vi "supercontinuumControl.vi"() -> ()   [LabVIEW 2011]
uses:
  monochromatorcontrol/perHandlemonochromator.vi
  users/nicolas/PHySpec-SDK-1.0.0/Labview-example/libPhyspec/libPhyspec.lvlib
panel:
  in  "readout rate (ms)":i32=2000 max=0
  in  "pm100usb":bool
  out "Laser power (µW)":dbl
  in  "RFonoff":bool
  in  "PortParameters":T1={"OpenPort"=TRUE, "ClosePort"=FALSE, "Baudrate"=115200, "Wait"=50, "ReadWrite"=FALSE}
  in  "InParameters":T2={"Destination"=18, "Source"=162, "Register"=144, "Array"=[], "WriteNotRead"=FALSE, "ReadWithPreample"=FALSE, "Ring"=3, "String"="", "Long"=0} {"Ring" items=["ByteArray", "IntegerArray", "String", "Long", "Direct string sent"]; "Register" format="%x"}
  out "peHandle":u32
  out "final error":errorcluster
  in  "Amplitude\nCH3 (%)":dbl=800.0 min=800.0 max=1400.0 step=1.0 format="%#.3g"
  in  "CH3 (nm)":dbl=800.0 min=800.0 max=1400.0 step=1.0 format="%#.3g"
  in  "Amplitude\nCH2 (%)":dbl=800.0 min=0.0 max=1400.0 step=0.1 format="%#.3g"
  in  "CH2 (nm)":dbl=800.0 min=800.0 max=1400.0 step=1.0 format="%#.3g"
  in  "Amplitude\nCH1 (%)":dbl=100.0 min=0.0 max=100.0 step=0.1 format="%#.3g"
  in  "CH1 (nm)":dbl=800.0 min=800.0 max=1400.0 step=1.0 format="%#.3g"
  in  "Amplitude\nCH0 (%)":dbl=100.0 min=0.0 max=100.0 step=0.1 format="%#.1f"
  in  "EXIT":bool
  in  "stop NKT  select":bool
  in  "CH0 (nm)":dbl=800.0 min=800.0 max=1400.0 step=1.0 format="%#.3g"
  in  "stop lttf":bool
  out "Current wavelength (nm)":dbl
  in  "SET wavelength (nm)":dbl max=0.0
  in  "NKT COM port":refnum<visa-resource-name>="COM21"
  out "NKT select":bool
  in  "NKT select start":bool
  out "LTTF contrast":bool
  in  "start LTTF filter":bool
  out "Fianium connected":bool
  in  "start fianium":bool
  out "Alarm":i32
  out "Output":string
  in  "Custom command":string
  out "Back Reflection Monitor":i32
  out "appended array":bool[](array[boolean])
  in  "100percent":bool
  in  "75percent":bool
  in  "50percent":bool
  in  "25percent":bool
  in  "power 0":bool
  in  "Set Power":i32 max=2100
  out "Power":i32
  out "Current Power":u8(slide) scale=0.0..100.0
  out "max Q":i32
  out "error out":errorcluster
  in  "Fianium COM port":refnum<visa-resource-name>="COM19"
  out "MachineState":string="init"
  in  "KEY":bool
  in  "stop fianium":bool
  # "Fianium WL-SC400 control"
  # "SET POWER"
  # "PM100"
  # "NKT Select"
  # "LTTF contrast"
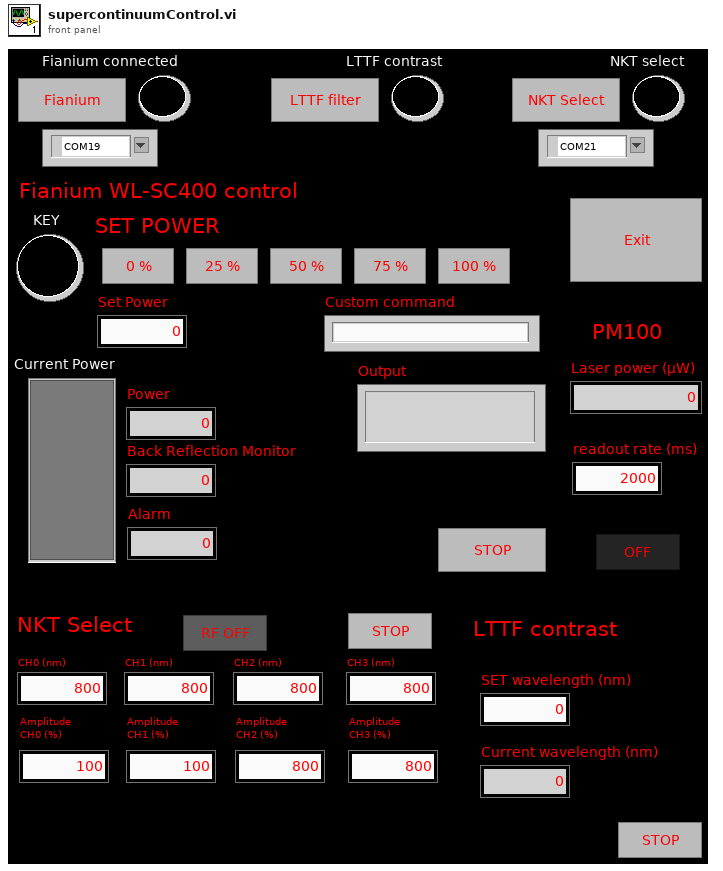
[diagram p1: front panel]
types:
  T1 = cluster{"OpenPort":bool, "ClosePort":bool, "Baudrate":i32, "Wait":u16, "ReadWrite":bool}
  T2 = cluster{"Destination":u8, "Source":u8, "Register":u8, "Array":i16[], "WriteNotRead":bool, "ReadWithPreample":bool, "Ring":u16, "String":string, "Long":i32}
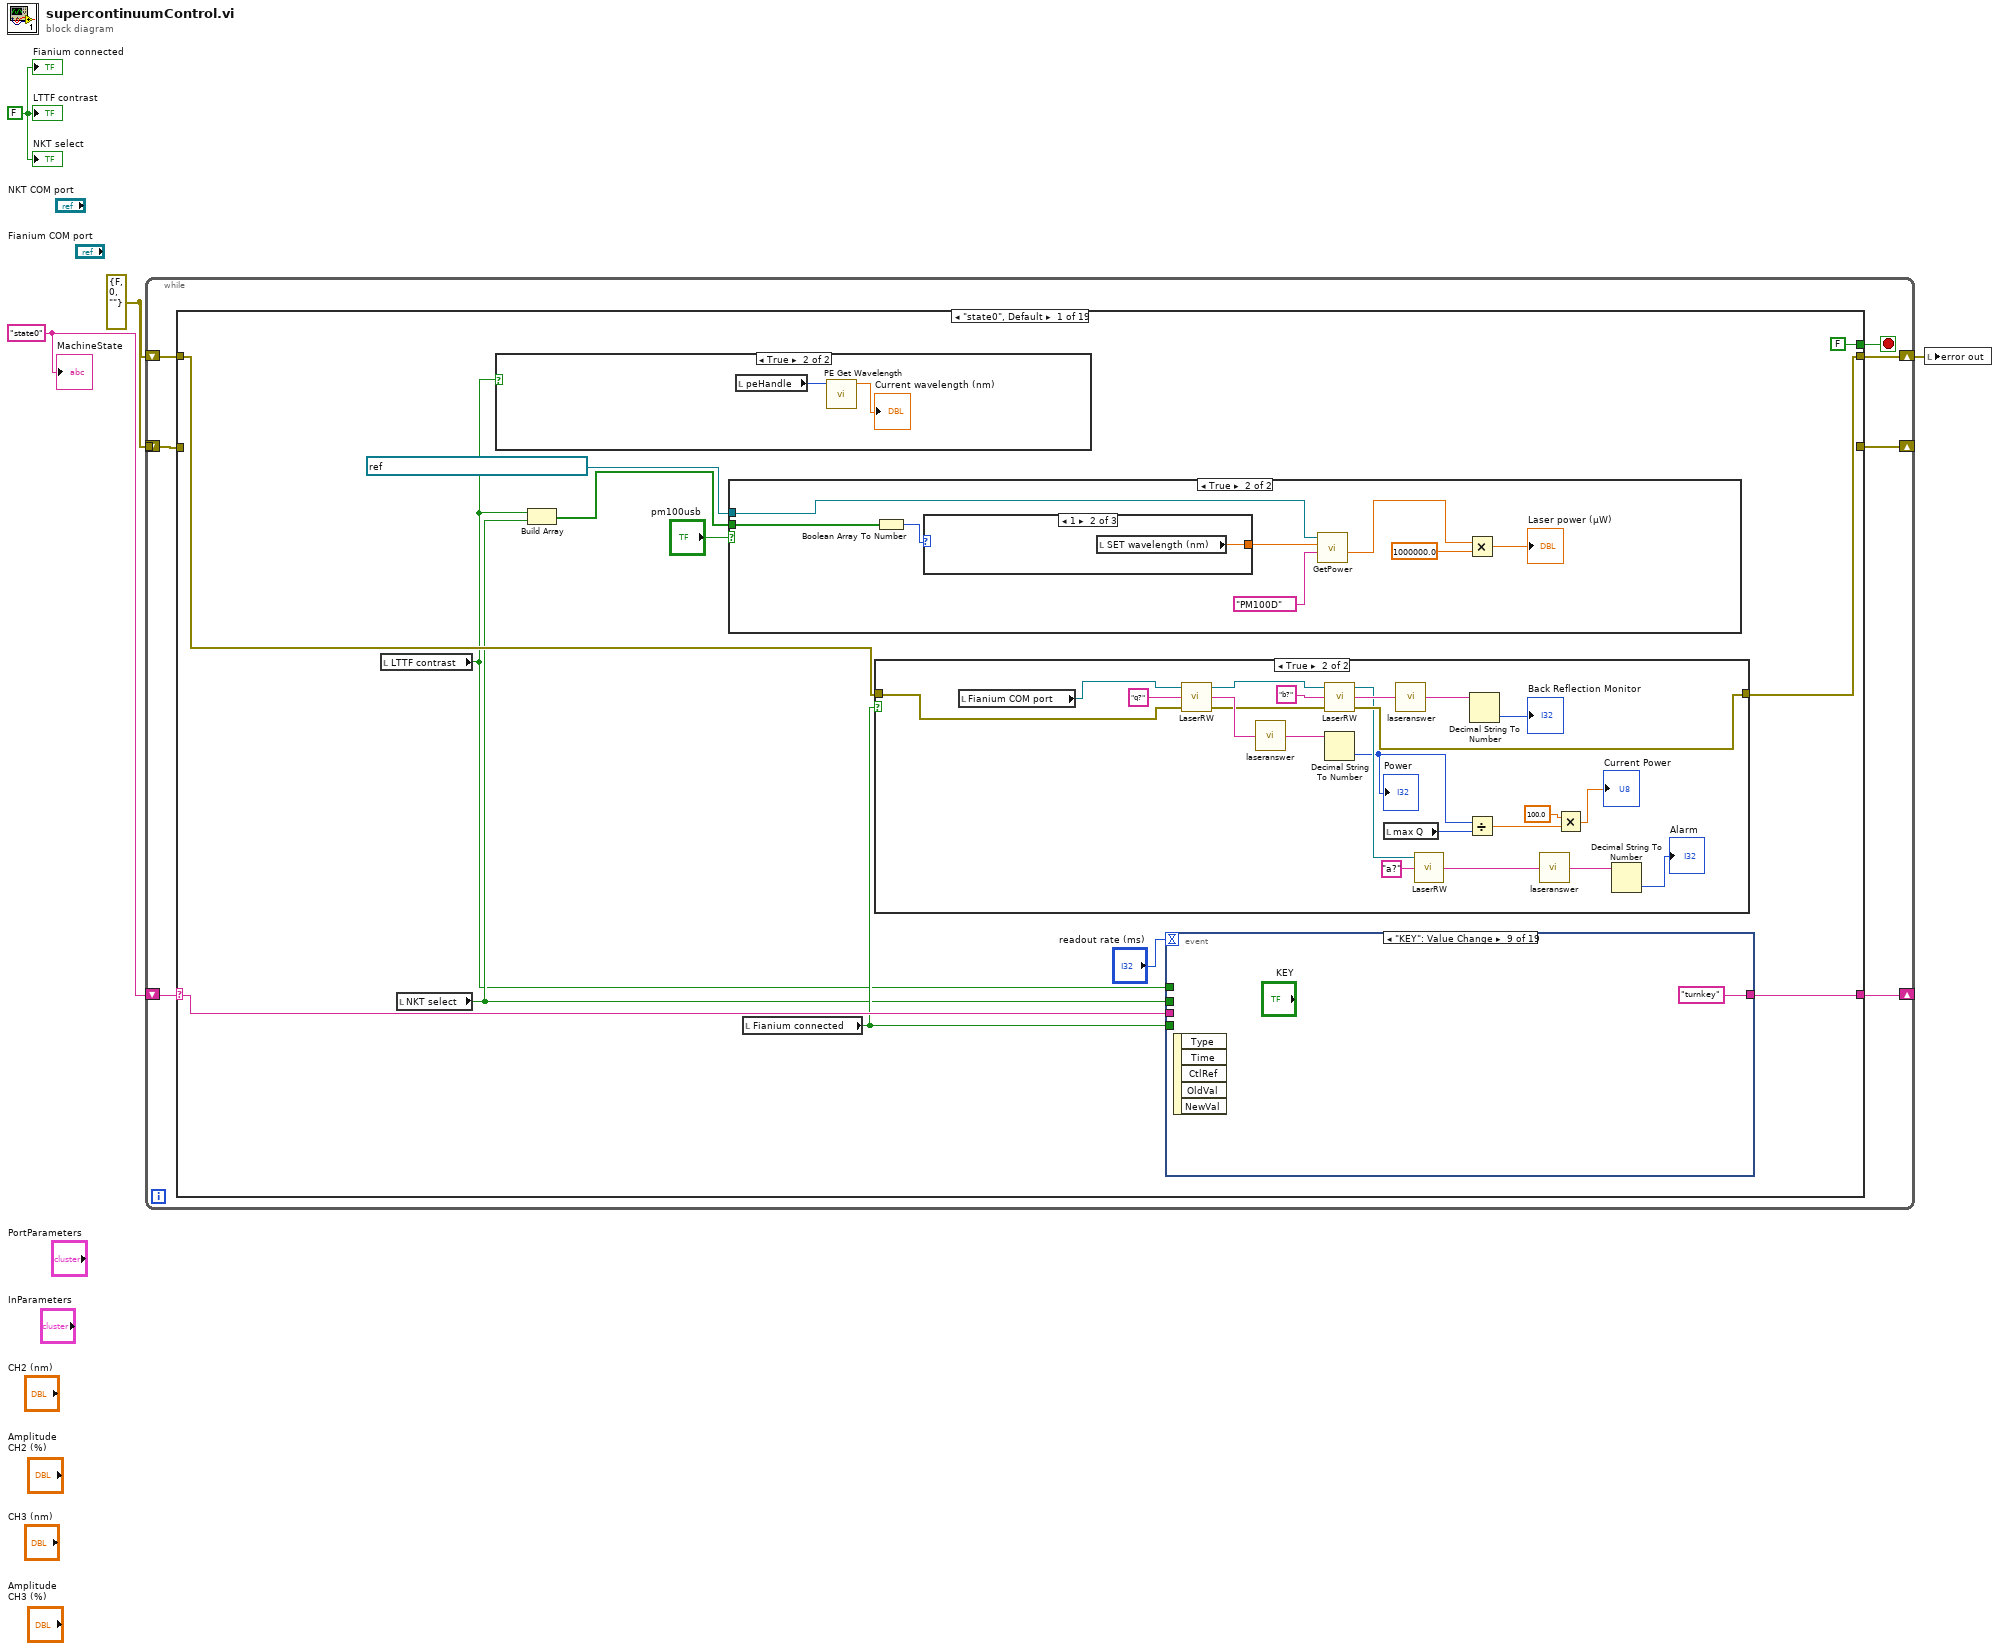
[diagram p0: block diagram]
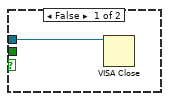
[diagram p2: hidden frame]
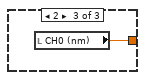
[diagram p4: hidden frame]
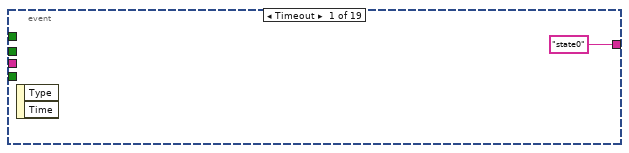
[diagram p7: hidden frame]
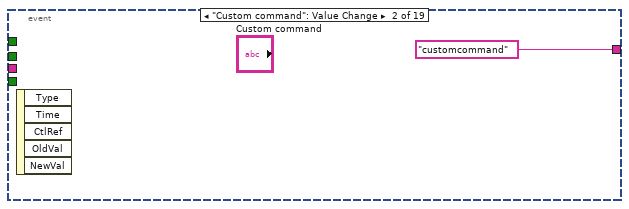
[diagram p8: hidden frame]
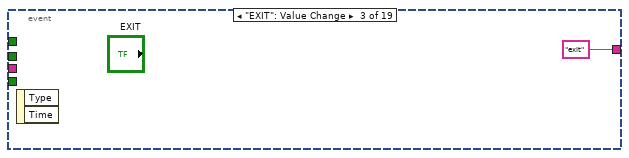
[diagram p9: hidden frame]
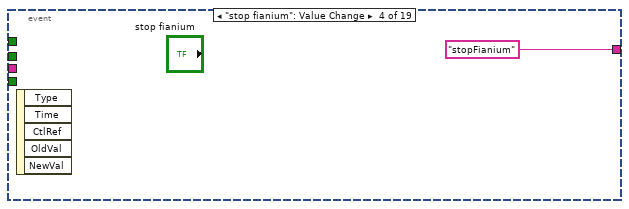
[diagram p10: hidden frame]
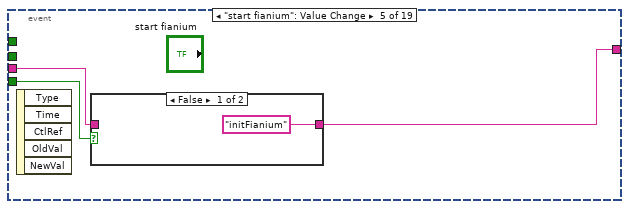
[diagram p11: hidden frame]
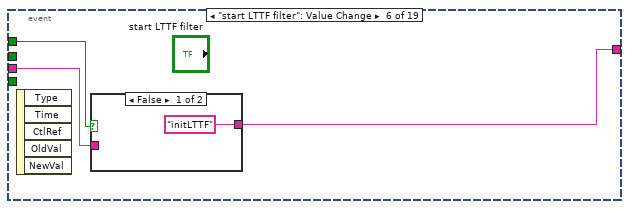
[diagram p13: hidden frame]
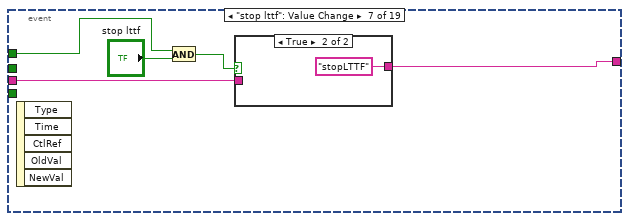
[diagram p15: hidden frame]
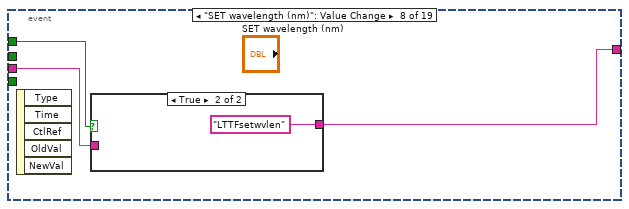
[diagram p17: hidden frame]
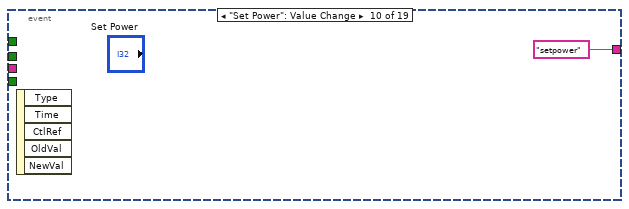
[diagram p19: hidden frame]
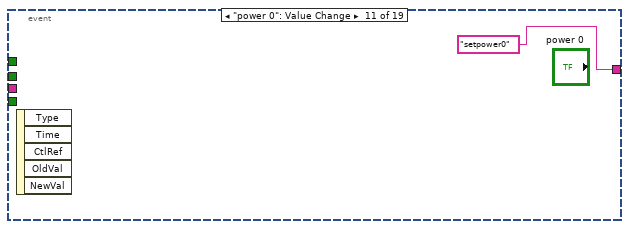
[diagram p20: hidden frame]
diagram:
  w2 = FALSE
  w1 = errorcluster {"status"=FALSE, "code"=0, "source"=""} ("error out")
  w4 = "state0"
  n1 = while {
    shift-right: [w10] -> _
    shift-left: w4 -> [w11]
    shift-right: [w8] -> w3
    shift-left: w1 -> [w7]
    shift-right: [w5] -> _
    shift-left: w1 -> [w6]
    tunnel: [w6] -> _
    stop <- w9 stop-if-true
    n2 = case shown="\"state0\", Default" w11 {
      selector: w11 -> [w19 _ _ _ _ _ _ _ _ _ _ _ _ _ _ _ _ _ _]
      tunnel: [w23 "state0" "state0" "state0" "" "state0" "state0" "state0" "state0" "state0" "state0" "state0" "state0" "state0" "state0" "state0" "state0" "state0" "state0"] -> w10
      tunnel: [FALSE _ _ _ TRUE FALSE FALSE FALSE FALSE FALSE _ FALSE _ _ _ _ _ _ _] -> w9
      tunnel: [w21 _ _ _ w167 w172 w180 w211 w216 w225 w244 w265 w282 w293 w302 w318 w335 w352 w378] -> w8
      tunnel: w7 -> [w22 _ _ _ w167 w173 w179 w212 w223 w227 w248 w267 w282 w293 w302 w318 w335 w352 w378]
      tunnel: w6 -> [_ w130 w149 w157 _ _ _ _ _ _ _ _ _ _ _ _ _ _ _]
      tunnel: [_ w131 w148 w156 _ _ _ _ _ _ _ _ _ _ _ _ _ _ _] -> w5
      frame "state0", Default {
        n3 = local read "LTTF contrast"() -> (w15:bool)
        n4 = local read "NKT select"() -> (w16:bool)
        n5 = case shown="True" w15 {
          frame False {
          }
          frame True {
            n6 = local read "peHandle"() -> (w35:u32)
            n7 = call "PE Get Wavelength.vi"("peHandle"=w35) -> ("wavelength"=→"Current wavelength (nm)":dbl)  [unwired: 8 in, 2 out]
          }
        }
        n8 = Build Array(w15, w16) -> (w13:bool[])
        n9 = case shown="True" "pm100usb" {
          tunnel: refnum<visa-resource-name> "USB0::0x1313::0x8072::P2007928::INSTR" ("Input Device") -> [w24 w31]
          tunnel: w13 -> [_ w28]
          frame False {
            n10 = VISA Close(VISA resource name=w24) -> ()  [unwired: 1 in, 1 out]
          }
          frame True {
            n11 = Boolean Array To Number(Boolean array=w28) -> (number=w27:u32)
            n12 = case shown="1" w27 {
              tunnel: [_ w33 w34] -> w26
              frame 0, Default {
              }
              frame 1 {
                n13 = local read "SET wavelength (nm)"() -> (w33:dbl)
              }
              frame 2 {
                n14 = local read "CH0 (nm)"() -> (w34:dbl)
              }
            }
            n15 = call "GetPower.vi"("Measeaurement mode"="PM100D", "Wavelength (nm)"=w26, "Input Device"=w31) -> ("Power (W)"=w30:dbl)  [unwired: 1 in, 3 out]
            n16 = Multiply(x=w30, y=1000000.0) -> (x*y=→"Laser power (µW)":dbl)
          }
        }
        n17 = local read "Fianium connected"() -> (w18:bool)
        n18 = case shown="True" w18 {
          tunnel: w22 -> [w37 w58]
          tunnel: [w37 w46] -> w21
          frame False {
          }
          frame True {
            n19 = local read "Fianium COM port"() -> (w59:refnum<visa-resource-name>)
            n20 = call "LaserRW.vi"("error in (no error)"=w58, "buffer à écrire"="q?", "Nom de ressource VISA"=w59) -> ("error out"=w49:errorcluster, "buffer lu"=w56:string, "Nom de ressource VISA en sortie"=w50:refnum<visa-resource-name>)
            n21 = call "laseranswer.vi"("IN"=w56) -> ("Answer"=w55:string)
            n22 = call "LaserRW.vi"("error in (no error)"=w49, "buffer à écrire"="b?", "Nom de ressource VISA"=w50) -> ("error out"=w46:errorcluster, "buffer lu"=w47:string, "Nom de ressource VISA en sortie"=w44:refnum<visa-resource-name>)
            n23 = Decimal String To Number(string=w55) -> (number=w39:i32)  [unwired: 2 in, 1 out]
            "Power" <- w39
            n24 = local read "max Q"() -> (w54:i32)
            n25 = call "laseranswer.vi"("IN"=w47) -> ("Answer"=w45:string)
            n26 = call "LaserRW.vi"("buffer à écrire"="a?", "Nom de ressource VISA"=w44) -> ("buffer lu"=w38:string)  [unwired: 1 in, 2 out]
            n27 = Divide(x=w39, y=w54) -> (x/y=w53:dbl)
            n28 = Decimal String To Number(string=w45) -> (number=→"Back Reflection Monitor":i32)  [unwired: 2 in, 1 out]
            n29 = call "laseranswer.vi"("IN"=w38) -> ("Answer"=w43:string)
            n30 = Multiply(x=100.0, y=w53) -> (x*y=→"Current Power":dbl)
            n31 = Decimal String To Number(string=w43) -> (number=→"Alarm":i32)  [unwired: 2 in, 1 out]
          }
        }
        n32 = event shown="[8] \"KEY\": Value Change" {
          selector: _ -> [_ _ _ _ _ _ _ _ _ _ _ _ _ _ _ _ _ _ _]
          dyn-events: _ -> [_ _ _ _ _ _ _ _ _ _ _ _ _ _ _ _ _ _ _]
          timeout: "readout rate (ms)" -> [_ _ _ _ _ _ _ _ _ _ _ _ _ _ _ _ _ _ _]
          tunnel: ["state0" "customcommand" "exit" "stopFianium" w66 w71 w78 w82 "turnkey" "setpower" "setpower0" "percentchange" w96 w102 w106 w112 w116 w121 w126] -> w23
          tunnel: w19 -> [_ _ _ _ w65 w70 w77 w81 _ _ _ _ w95 w101 w105 w110 w115 w120 w125]
          tunnel: w18 -> [_ _ _ _ w64 _ _ _ _ _ _ _ _ _ _ _ _ _ _]
          tunnel: w15 -> [_ _ _ _ _ w69 w75 w83 _ _ _ _ _ _ _ _ _ _ _]
          tunnel: w16 -> [_ _ _ _ _ _ _ _ _ _ _ _ w97 w100 w107 w111 w117 w122 w127]
          event Timeout {
            n33 = event-data() -> ()  [unwired: 1 in, 2 out]
          }
          event "Custom command": Value Change {
            n34 = event-data() -> ()  [unwired: 1 in, 5 out]
          }
          event "EXIT": Value Change {
            n35 = event-data() -> ()  [unwired: 1 in, 2 out]
          }
          event "stop fianium": Value Change {
            n36 = event-data() -> ()  [unwired: 1 in, 5 out]
          }
          event "start fianium": Value Change {
            n37 = event-data() -> ()  [unwired: 1 in, 5 out]
            n38 = case shown="False" w64 {
              tunnel: ["initFianium" w68] -> w66
              tunnel: w65 -> [_ w68]
              frame False {
              }
              frame True {
              }
            }
          }
          event "start LTTF filter": Value Change {
            n39 = event-data() -> ()  [unwired: 1 in, 5 out]
            n40 = case shown="False" w69 {
              tunnel: ["initLTTF" w73] -> w71
              tunnel: w70 -> [_ w73]
              frame False {
              }
              frame True {
              }
            }
          }
          event "stop lttf": Value Change {
            n41 = event-data() -> ()  [unwired: 1 in, 5 out]
            n42 = And(x=w75, y="stop lttf") -> (x .and. y?=w74:bool)
            n43 = case shown="True" w74 {
              tunnel: [w79 "stopLTTF"] -> w78
              tunnel: w77 -> [w79 _]
              frame False {
              }
              frame True {
              }
            }
          }
          event "SET wavelength (nm)": Value Change {
            n44 = event-data() -> ()  [unwired: 1 in, 5 out]
            n45 = case shown="True" w83 {
              tunnel: [w84 "LTTFsetwvlen"] -> w82
              tunnel: w81 -> [w84 _]
              frame False {
              }
              frame True {
              }
            }
          }
          event "KEY": Value Change {
            n46 = event-data() -> ()  [unwired: 1 in, 5 out]
          }
          event "Set Power": Value Change {
            n47 = event-data() -> ()  [unwired: 1 in, 5 out]
          }
          event "power 0": Value Change {
            n48 = event-data() -> ()  [unwired: 1 in, 5 out]
          }
          event "25percent", "50percent", "75percent", "100percent": Value Change {
            n49 = event-data() -> ()  [unwired: 1 in, 5 out]
            n50 = Build Array("25percent", "50percent", "75percent", "100percent") -> (→"appended array":bool[])
          }
          event "NKT select start": Value Change {
            n51 = event-data() -> ()  [unwired: 1 in, 5 out]
            n52 = case shown="False" w97 {
              tunnel: ["NKTSELECTstart" w99] -> w96
              tunnel: w95 -> [_ w99]
              frame False {
              }
              frame True {
              }
            }
          }
          event "stop NKT  select": Value Change {
            n53 = event-data() -> ()  [unwired: 1 in, 5 out]
            n54 = case shown="True" w100 {
              tunnel: w101 -> [w103 _]
              tunnel: [w103 "NKTSELECTstop"] -> w102
              frame False {
              }
              frame True {
              }
            }
          }
          event "CH0 (nm)": Value Change {
            n55 = event-data() -> ()  [unwired: 1 in, 7 out]
            n56 = case shown="True" w107 {
              tunnel: [w108 "NKTSELECTch0wv"] -> w106
              tunnel: w105 -> [w108 _]
              frame False {
              }
              frame True {
              }
            }
          }
          event "Amplitude\nCH0 (%)": Value Change {
            n57 = event-data() -> ()  [unwired: 1 in, 5 out]
            n58 = case shown="True" w111 {
              tunnel: [w113 "NKTSELECTampch0"] -> w112
              tunnel: w110 -> [w113 _]
              frame False {
              }
              frame True {
              }
            }
          }
          event "RFonoff": Value Change {
            n59 = event-data() -> ()  [unwired: 1 in, 5 out]
            n60 = case shown="False" w117 {
              tunnel: [w118 "NKTselectrfonoff"] -> w116
              tunnel: w115 -> [w118 _]
              frame False {
              }
              frame True {
              }
            }
          }
          event "CH1 (nm)": Value Change {
            n61 = event-data() -> ()  [unwired: 1 in, 5 out]
            n62 = case shown="True" w122 {
              tunnel: [w123 "NKTSELECTch1wv"] -> w121
              tunnel: w120 -> [w123 _]
              frame False {
              }
              frame True {
              }
            }
          }
          event "Amplitude\nCH1 (%)": Value Change {
            n63 = event-data() -> ()  [unwired: 1 in, 5 out]
            n64 = case shown="True" w127 {
              tunnel: [w128 "NKTSELECTampch1"] -> w126
              tunnel: w125 -> [w128 _]
              frame False {
              }
              frame True {
              }
            }
          }
        }
      }
      frame "initLTTF" {
        n65 = Path To String(path=path "C:/Program Files (x86)/Photon etc/PHySpecV2/system.xml" ("Configuration File")) -> (string=w136:string)
        n66 = call "PE Create.vi"("error in (no error)"=w130, "conffile"=w136) -> ("error out"=w138:errorcluster, "peHandle"=w137:u32)  [unwired: 7 in, 1 out]
        n67 = case shown="No Error" w138 {
          selector: w138 -> [w144 w147]
          tunnel: w137 -> [w141 _]
          tunnel: [w141 _] -> w134
          tunnel: [w140 w147] -> w131
          frame No Error {
            n68 = call "PE Get System Name.vi"("error in (no error)"=w144, "size"=4095, "index"=0, "peHandle"=w141) -> ("error out"=w143:errorcluster, "name"=w142:string)  [unwired: 5 in, 1 out]
            n69 = call "PE Open.vi"("error in (no error)"=w143, "name"=w142, "peHandle"=w141) -> ("error out"=w140:errorcluster)  [unwired: 7 in, 1 out]
          }
          frame Error {
          }
        }
        "peHandle" <- w134
        n70 = global write "perHandlemonochromator.vi" "peHandle"(w134) -> ()
        n71 = Unbundle By Name(w131) -> ("status"=w133:bool)
        n72 = Not(x=w133) -> (.not. x?=w132:bool)
        n73 = local write "LTTF contrast"(w132) -> ()
      }
      frame "LTTFsetwvlen" {
        n74 = local read "SET wavelength (nm)"() -> (w152:dbl)
        n75 = In Range and Coerce(upper limit=400.0, x=w152, lower limit=1100.0) -> (coerced(x)=w151:dbl)  [unwired: 1 out]
        n76 = local read "peHandle"() -> (w150:u32)
        n77 = call "PE Set Wavelength.vi"("error in (no error)"=w149, "wavelength"=w151, "peHandle"=w150) -> ("error out"=w148:errorcluster)  [unwired: 7 in, 1 out]
      }
      frame "stopLTTF" {
        n78 = local write "LTTF contrast"(FALSE) -> ()
        n79 = case shown="No Error" w157 {
          selector: w157 -> [w161 w164]
          tunnel: [w160 w164] -> w156
          frame No Error {
            n80 = local read "peHandle"() -> (w162:u32)
            n81 = call "PE Close.vi"("error in (no error)"=w161, "peHandle"=w162) -> ("error out"=w163:errorcluster)  [unwired: 8 in, 1 out]
            n82 = call "PE Destroy.vi"("error in (no error)"=w163, "peHandle"=w162) -> ("error out"=w160:errorcluster)  [unwired: 8 in, 1 out]
          }
          frame Error {
          }
        }
      }
      frame "exit" {
      }
      frame "customcommand" {
        n83 = local read "Custom command"() -> (w174:string)
        n84 = local read "Fianium COM port"() -> (w170:refnum<visa-resource-name>)
        n85 = call "LaserRW.vi"("error in (no error)"=w173, "buffer à écrire"=w174, "Nom de ressource VISA"=w170) -> ("error out"=w172:errorcluster, "buffer lu"=→"Output":string)  [unwired: 1 out]
      }
      frame "percentchange" {
        n86 = local read "appended array"() -> (w185:bool[])
        n87 = Boolean Array To Number(Boolean array=w185) -> (number=w176:u32)
        n88 = local read "max Q"() -> (w184:i32)
        n89 = case shown="1" w176 {
          tunnel: w184 -> [_ w193 w197 w202 w207]
          tunnel: [0.0 w194 w198 w201 w205] -> w177
          frame 0, Default {
          }
          frame 2 {
            n90 = Multiply(x=0.5, y=w193) -> (x*y=w195:dbl)
            n91 = Round Toward -Infinity(1:w195) -> (0:w194:dbl)
          }
          frame 4 {
            n92 = Multiply(x=0.75, y=w197) -> (x*y=w199:dbl)
            n93 = Round Toward -Infinity(1:w199) -> (0:w198:dbl)
          }
          frame 8 {
            n94 = Multiply(x=1, y=w202) -> (x*y=w203:i32)
            n95 = Round Toward -Infinity(1:w203) -> (0:w201:i32)
          }
          frame 1 {
            n96 = Multiply(x=0.25, y=w207) -> (x*y=w206:dbl)
            n97 = Round Toward -Infinity(1:w206) -> (0:w205:dbl)
          }
        }
        n98 = Number To Decimal String(number=w177) -> (decimal integer string=w183:string)  [unwired: 1 in]
        n99 = local read "Fianium COM port"() -> (w178:refnum<visa-resource-name>)
        n100 = Concatenate Strings("q=" ("string"), w183) -> (w181:string)
        n101 = case shown="0" w176 {
          tunnel: w181 -> [_ w191]
          tunnel: [w187 w190] -> w180
          tunnel: w179 -> [w187 w189]
          tunnel: w178 -> [_ w188]
          frame 0 {
          }
          frame 1, Default {
            n102 = call "LaserRW.vi"("error in (no error)"=w189, "buffer à écrire"=w191, "Nom de ressource VISA"=w188) -> ("error out"=w190:errorcluster)  [unwired: 2 out]
          }
        }
      }
      frame "setpower0" {
        n103 = local read "Fianium COM port"() -> (w213:refnum<visa-resource-name>)
        n104 = call "LaserRW.vi"("error in (no error)"=w212, "buffer à écrire"="q=0", "Nom de ressource VISA"=w213) -> ("error out"=w211:errorcluster)  [unwired: 2 out]
      }
      frame "setpower" {
        n105 = local read "Set Power"() -> (w222:i32)
        n106 = Number To Decimal String(number=w222) -> (decimal integer string=w221:string)  [unwired: 1 in]
        n107 = local read "Fianium COM port"() -> (w218:refnum<visa-resource-name>)
        n108 = Concatenate Strings("q=" ("string"), w221) -> (w219:string)
        n109 = call "LaserRW.vi"("error in (no error)"=w223, "buffer à écrire"=w219, "Nom de ressource VISA"=w218) -> ("error out"=w216:errorcluster)  [unwired: 2 out]
      }
      frame "turnkey" {
        n110 = local read "Fianium COM port"() -> (w229:refnum<visa-resource-name>)
        n111 = local read "KEY"() -> (w231:bool)
        n112 = case shown="False" w231 {
          tunnel: ["key=0" "key=1"] -> w230
          tunnel: w229 -> [w237 w239]
          tunnel: [w235 w239] -> w228
          tunnel: w227 -> [w234 w238]
          tunnel: [w234 w238] -> w226
          frame False {
            n113 = call "LaserRW.vi"("buffer à écrire"="q=0", "Nom de ressource VISA"=w237) -> ("Nom de ressource VISA en sortie"=w235:refnum<visa-resource-name>)  [unwired: 1 in, 2 out]
          }
          frame True {
          }
        }
        n114 = call "LaserRW.vi"("error in (no error)"=w226, "buffer à écrire"=w230, "Nom de ressource VISA"=w228) -> ("error out"=w225:errorcluster)  [unwired: 2 out]
      }
      frame "stopFianium" {
        n115 = local write "Fianium connected"(FALSE ("Fianium connected")) -> ()
        n116 = local read "Fianium COM port"() -> (w250:refnum<visa-resource-name>)
        n117 = local read "KEY"() -> (w249:bool)
        n118 = case shown="True" w249 {
          tunnel: w250 -> [w252 w261]
          tunnel: w248 -> [w253 w257]
          tunnel: [w253 w255] -> w247
          tunnel: [w252 w254] -> w246
          frame False {
          }
          frame True {
            n119 = call "LaserRW.vi"("error in (no error)"=w257, "buffer à écrire"="q=0", "Nom de ressource VISA"=w261) -> ("error out"=w256:errorcluster, "Nom de ressource VISA en sortie"=w258:refnum<visa-resource-name>)  [unwired: 1 out]
            n120 = call "LaserRW.vi"("error in (no error)"=w256, "buffer à écrire"="key=0", "Nom de ressource VISA"=w258) -> ("error out"=w255:errorcluster, "Nom de ressource VISA en sortie"=w254:refnum<visa-resource-name>)  [unwired: 1 out]
          }
        }
        n121 = call "LaserRW.vi"("error in (no error)"=w247, "buffer à écrire"="switch=0", "Nom de ressource VISA"=w246) -> ("error out"=w244:errorcluster, "Nom de ressource VISA en sortie"=w243:refnum<visa-resource-name>)  [unwired: 1 out]
        n122 = VISA Close(VISA resource name=w243) -> (error out=→"final error":errorcluster)  [unwired: 1 in]
      }
      frame "initFianium" {
        n123 = local write "Fianium connected"(TRUE ("Fianium connected")) -> ()
        n124 = local read "Fianium COM port"() -> (w264:refnum<visa-resource-name>)
        n125 = call "LaserRW.vi"("error in (no error)"=w267, "buffer à écrire"="x=2", "Nom de ressource VISA"=w264) -> ("error out"=w266:errorcluster, "Nom de ressource VISA en sortie"=w263:refnum<visa-resource-name>)  [unwired: 1 out]
        n126 = call "LaserRW.vi"("error in (no error)"=w266, "buffer à écrire"="s?", "Nom de ressource VISA"=w263) -> ("error out"=w268:errorcluster, "buffer lu"=w279:string, "Nom de ressource VISA en sortie"=w275:refnum<visa-resource-name>)
        "error out" <- w268
        n127 = call "LaserRW.vi"("error in (no error)"=w268, "buffer à écrire"="hwkey?", "Nom de ressource VISA"=w275) -> ("error out"=w265:errorcluster, "buffer lu"=w274:string)  [unwired: 1 out]
        n128 = call "laseranswer.vi"("IN"=w279) -> ("Answer"=w278:string)
        n129 = call "laseranswer.vi"("IN"=w274) -> ("Answer"=w272:string)
        n130 = Decimal String To Number(string=w278) -> (number=w277:i32)  [unwired: 2 in, 1 out]
        "max Q" <- w277
        n131 = Decimal String To Number(string=w272) -> (number=w271:i32)  [unwired: 2 in, 1 out]
        n132 = property on="Set Power" class="DigNum (strict)"("Maximum"=w277) -> ()  [unwired: 2 in, 2 out]
        n133 = Not Equal To 0?(x=w271) -> (x != 0?=w270:bool)
        n134 = local write "KEY"(w270) -> ()
      }
      frame "NKTSELECTstart" {
        w286 = FALSE
        n135 = local read "PortParameters"() -> (w289:T1)
        n136 = local read "NKT COM port"() -> (w290:refnum<visa-resource-name>)
        n137 = Bundle By Name(cluster=w289, "OpenPort"=TRUE, "ClosePort"=w286, "ReadWrite"=w286) -> (w288:T1)
        n138 = call "NGSerialPort_withreturn.vi"("PortParameters"=w288, "VISA in"=w290) -> ("error out"=w285:errorcluster)  [unwired: 6 in, 3 out]
        n139 = Unbundle By Name(w285) -> ("status"=w283:bool)
        n140 = Not(x=w283) -> (.not. x?=w284:bool)
        n141 = local write "NKT select"(w284) -> ()
      }
      frame "NKTSELECTstop" {
        w295 = FALSE
        n142 = local read "PortParameters"() -> (w299:T1)
        n143 = local read "NKT COM port"() -> (w296:refnum<visa-resource-name>)
        n144 = Bundle By Name(cluster=w299, "OpenPort"=w295, "ClosePort"=TRUE, "ReadWrite"=w295) -> (w297:T1)
        n145 = local write "NKT select"(w295) -> ()
        n146 = call "NGSerialPort_withreturn.vi"("PortParameters"=w297, "VISA in"=w296) -> ("VISA out"=w292:refnum<visa-resource-name>)  [unwired: 6 in, 3 out]
        n147 = VISA Close(VISA resource name=w292) -> ()  [unwired: 1 in, 1 out]
      }
      frame "NKTSELECTch0wv" {
        w314 = FALSE
        w313 = TRUE
        n148 = local read "CH0 (nm)"() -> (w312:dbl)
        n149 = Multiply(x=w312, y=1000.0) -> (x*y=w310:dbl)
        n150 = local read "PortParameters"() -> (w315:T1)
        n151 = local read "InParameters"() -> (w316:T2)
        n152 = To Unsigned Long Integer(number=w310) -> (unsigned 32bit integer=w309:u32)
        n153 = local read "NKT COM port"() -> (w305:refnum<visa-resource-name>)
        n154 = Bundle By Name(cluster=w316, "Destination"=u8 18, "Source"=u8 162, "Register"=u8 144, "Long"=w309, "WriteNotRead"=w313, "Ring"=u16 3) -> (w304:T2)
        n155 = Bundle By Name(cluster=w315, "OpenPort"=w314, "ClosePort"=w314, "ReadWrite"=w313) -> (w303:T1)
        n156 = call "NGSerialPort_withreturn.vi"("PortParameters"=w303, "InParameters"=w304, "VISA in"=w305) -> ()  [unwired: 5 in, 4 out]
      }
      frame "NKTSELECTch1wv" {
        w330 = FALSE
        w329 = TRUE
        n157 = local read "CH1 (nm)"() -> (w328:dbl)
        n158 = Multiply(x=w328, y=1000.0) -> (x*y=w326:dbl)
        n159 = local read "PortParameters"() -> (w331:T1)
        n160 = local read "InParameters"() -> (w332:T2)
        n161 = To Unsigned Long Integer(number=w326) -> (unsigned 32bit integer=w325:u32)
        n162 = local read "NKT COM port"() -> (w321:refnum<visa-resource-name>)
        n163 = Bundle By Name(cluster=w332, "Destination"=u8 18, "Source"=u8 162, "Register"=u8 145, "Long"=w325, "WriteNotRead"=w329) -> (w320:T2)
        n164 = Bundle By Name(cluster=w331, "OpenPort"=w330, "ClosePort"=w330, "ReadWrite"=w329) -> (w319:T1)
        n165 = call "NGSerialPort_withreturn.vi"("PortParameters"=w319, "InParameters"=w320, "VISA in"=w321) -> ()  [unwired: 5 in, 4 out]
      }
      frame "NKTSELECTampch0" {
        w347 = FALSE
        w346 = TRUE
        n166 = local read "Amplitude\nCH0 (%)"() -> (w345:dbl)
        n167 = Multiply(x=w345, y=10.0) -> (x*y=w343:dbl)
        n168 = local read "PortParameters"() -> (w348:T1)
        n169 = local read "InParameters"() -> (w349:T2)
        n170 = To Unsigned Long Integer(number=w343) -> (unsigned 32bit integer=w342:u32)
        n171 = local read "NKT COM port"() -> (w338:refnum<visa-resource-name>)
        n172 = Bundle By Name(cluster=w349, "Destination"=u8 18, "Source"=u8 162, "Register"=u8 176, "Long"=w342, "WriteNotRead"=w346, "Ring"=u16 3) -> (w337:T2)
        n173 = Bundle By Name(cluster=w348, "OpenPort"=w347, "ClosePort"=w347, "ReadWrite"=w346) -> (w336:T1)
        n174 = call "NGSerialPort_withreturn.vi"("PortParameters"=w336, "InParameters"=w337, "VISA in"=w338) -> ()  [unwired: 5 in, 4 out]
      }
      frame "NKTSELECTampch1" {
        w364 = FALSE
        w363 = TRUE
        n175 = local read "Amplitude\nCH1 (%)"() -> (w362:dbl)
        n176 = Multiply(x=w362, y=10.0) -> (x*y=w360:dbl)
        n177 = local read "PortParameters"() -> (w365:T1)
        n178 = local read "InParameters"() -> (w366:T2)
        n179 = To Unsigned Long Integer(number=w360) -> (unsigned 32bit integer=w359:u32)
        n180 = local read "NKT COM port"() -> (w355:refnum<visa-resource-name>)
        n181 = Bundle By Name(cluster=w366, "Destination"=u8 18, "Source"=u8 162, "Register"=u8 177, "Long"=w359, "WriteNotRead"=w363, "Ring"=u16 3) -> (w354:T2)
        n182 = Bundle By Name(cluster=w365, "OpenPort"=w364, "ClosePort"=w364, "ReadWrite"=w363) -> (w353:T1)
        n183 = call "NGSerialPort_withreturn.vi"("PortParameters"=w353, "InParameters"=w354, "VISA in"=w355) -> ()  [unwired: 5 in, 4 out]
      }
      frame "NKTselectrfonoff" {
        w385 = FALSE
        w384 = TRUE
        n184 = local read "RFonoff"() -> (w376:bool)
        n185 = Boolean To (0,1)(Boolean=w376) -> (0, 1=w374:i16)
        n186 = local read "InParameters"() -> (w375:T2)
        n187 = Build Array(w374) -> (w373:i16[])
        n188 = local read "PortParameters"() -> (w386:T1)
        n189 = Bundle By Name(cluster=w375, "Destination"=u8 18, "Source"=u8 162, "Register"=u8 48, "Array"=w373, "WriteNotRead"=w384, "Ring"=u16 1) -> (w371:T2)
        n190 = local read "NKT COM port"() -> (w380:refnum<visa-resource-name>)
        n191 = Bundle By Name(cluster=w386, "OpenPort"=w385, "ClosePort"=w385, "ReadWrite"=w384) -> (w379:T1)
        n192 = Bundle By Name(cluster=w371, "Destination"=u8 16) -> (w369:T2)
        n193 = call "NGSerialPort_withreturn.vi"("PortParameters"=w379, "InParameters"=w371, "VISA in"=w380) -> ("VISA out"=w367:refnum<visa-resource-name>, "PortParameters OUT"=w368:T1)  [unwired: 5 in, 2 out]
        n194 = call "NGSerialPort_withreturn.vi"("PortParameters"=w368, "InParameters"=w369, "VISA in"=w367) -> ()  [unwired: 5 in, 4 out]
      }
    }
  }
  n195 = local write "error out"(w3) -> ()
  "MachineState" <- w4
  "Fianium connected" <- w2
  "LTTF contrast" <- w2
  "NKT select" <- w2
